vi "Create Force Accuracy Test Waveform.vi"(11 "Model in":refnum<class "Model.lvclass">) -> (2 "Waveform":refnum<class "Waveform.lvclass">, 3 "Model out":refnum<class "Model.lvclass">)   [LabVIEW 2016]
uses:
  Typedefs/WaveformTypes.ctl
  Typedefs/WaveformSettings.ctl
  Model/Waveforms/Waveform Factory/Waveform Factory.lvclass
  Model/Model/Model.lvclass
  Model/Waveforms/Waveform/Waveform.lvclass
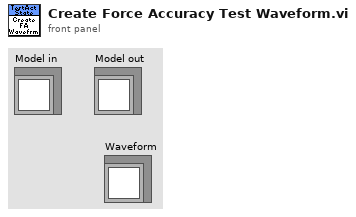
[diagram p1: front panel]
types:
  T1 = typedef "WaveformTypes.ctl" = enum16{"Sine", "Triangle", "Square", "Sawtooth", "Chirp", "Gaussian", "Trapezoid", "Constant"}
  T2 = typedef "WaveformSettings.ctl" = cluster{"Sample Count":u32, "Amplitude":dbl, "Offset":dbl, "Frequency":dbl[unit], "Waveform":T1, "F1":dbl[unit], "F2":dbl[unit], "Duty Cycle":dbl, "ILC Rate":dbl[unit], "Ramp Time":dbl[unit], "Hold Time":dbl[unit], "Settling Time":dbl[unit], "Delay":dbl[unit]}
  T3 = typedef "ForceAccuracyTestSettings.ctl" = cluster{"Max Force Error (N)":dbl, "Max Moment (NM)":dbl, "Process Time (s)":dbl, "Sample Time (s)":dbl, "Iterations":i32, "Amplitude (N)":dbl, "Non-Repeating Error":dbl}
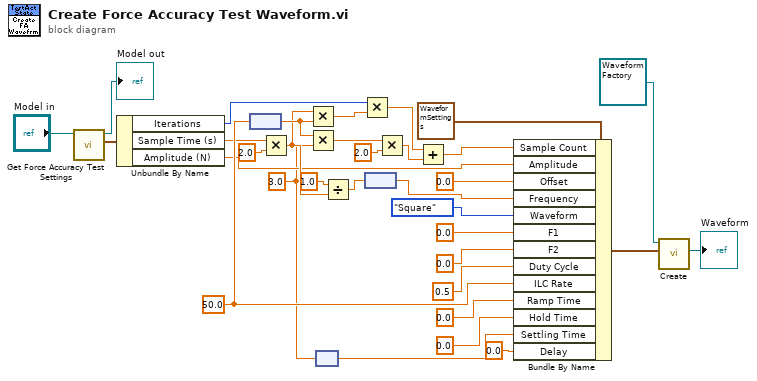
[diagram p0: block diagram]
diagram:
  w1 = 3.0
  w26 = dbl[unit] 50.0 ("ILC Rate")
  n1 = call-dynamic "Get Force Accuracy Test Settings.vi"("Model in"="Model in") -> ("Force Accuracy Test Settings"=w13:T3, "Model out"=→"Model out":refnum<class "Model.lvclass">)  [unwired: 9 in]
  n2 = Unbundle By Name(w13) -> ("Iterations"=w4:i32, "Sample Time (s)"=w6:dbl, "Amplitude (N)"=w14:dbl)
  n3 = node(w26) -> (w28:dbl)
  n4 = Multiply(x=w6, y=2.0) -> (x*y=w27:dbl)
  n5 = Multiply(x=w27, y=w28) -> (x*y=w3:dbl)
  n6 = Multiply(x=w28, y=w1) -> (x*y=w29:dbl)
  n7 = node(w1) -> (w5:dbl[unit])
  n8 = Divide(x=1.0, y=w27) -> (x/y=w24:dbl)
  n9 = Multiply(x=w4, y=w3) -> (x*y=w2:dbl)
  n10 = node(w24) -> (w25:dbl[unit])
  n11 = Multiply(x=w29, y=2.0) -> (x*y=w31:dbl)
  n12 = Add(x=w2, y=w31) -> (x+y=w32:dbl)
  n13 = Bundle By Name(cluster=T2 {"Sample Count"=0, "Amplitude"=0.0, "Offset"=0.0, "Frequency"=0.0, "Waveform"=enum."Sine", "F1"=0.0, "F2"=0.0, "Duty Cycle"=0.0, "ILC Rate"=0.0, "Ramp Time"=0.0, "Hold Time"=0.0, "Settling Time"=0.0, "Delay"=0.0} ("Waveform Settings"), "Sample Count"=w32, "Amplitude"=w14, "Offset"=0.0, "Frequency"=w25, "Waveform"=WaveformTypes."Square", "F1"=dbl[unit] 0.0, "F2"=dbl[unit] 0.0, "Duty Cycle"=0.5, "ILC Rate"=w26, "Ramp Time"=dbl[unit] 0.0, "Hold Time"=dbl[unit] 0.0, "Settling Time"=w5, "Delay"=dbl[unit] 0.0) -> (w8:T2)
  n14 = call-dynamic "Create.vi"("Waveform Settings"=w8, "Waveform Factory in"=refnum<class "Waveform Factory.lvclass"> refnum ("Waveform Factory.lvclass")) -> ("Waveform"=→"Waveform":refnum<class "Waveform.lvclass">)  [unwired: 7 in, 2 out]
